vi "disdrometer_distrubitons.vi"(10 "Spectrum Vector":dbl[](array[numeric])=[1.0, 2.0, 3.0, 4.0, 5.0, 6.0, 7.0, 8.0, 9.0, 10.0, 11.0, 12.0]) -> (0 "Velocity Distribution":dbl[](array[numeric]), 1 "Diameter Distribution":dbl[](array[numeric]), 2 "Distribution Matrix":dbl[][](array[numeric]))   [LabVIEW 2018]
doc: "Separates disdrometer spectrum data into a diameter distribution array and a speed distribution array."
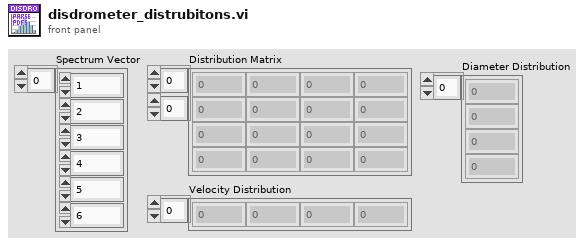
[diagram p1: front panel]
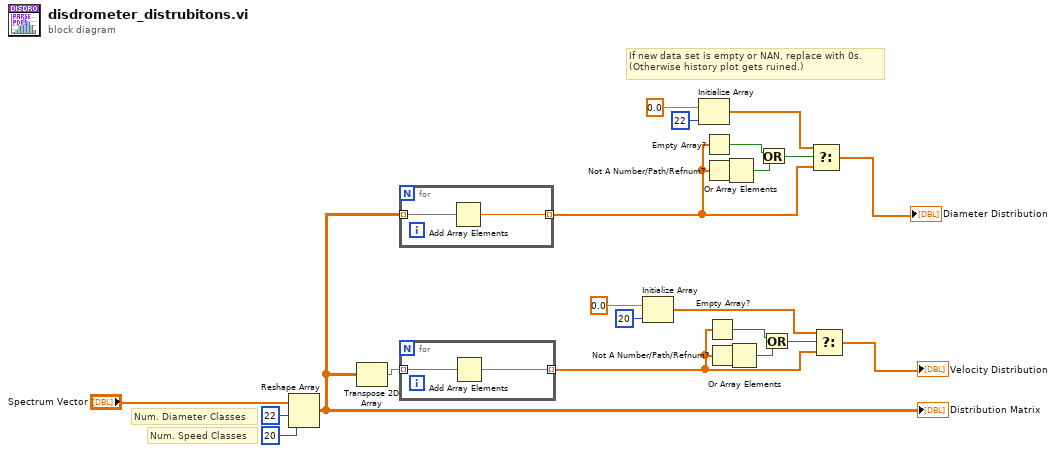
[diagram p0: block diagram]
diagram:
  # "If new data set is empty or NAN, replace with 0s.\n(Otherwise history plot gets ruined.)"
  # "Num. Speed Classes"
  # "Num. Diameter Classes"
  n1 = Reshape Array("Spectrum Vector", 22 ("dimension size"), 20 ("dimension size")) -> (w19:dbl[][])
  "Distribution Matrix" <- w19
  n2 = Transpose 2D Array(2D array=w19) -> (transposed array=w21:dbl[][])
  n3 = for {
    tunnel: w19 -> [w25] mode=indexing
    tunnel: [w24] -> w9 mode=indexing
    n4 = Add Array Elements(numeric array=w25) -> (sum=w24:dbl)
  }
  n5 = for {
    tunnel: w21 -> [w27] mode=indexing
    tunnel: [w26] -> w3 mode=indexing
    n6 = Add Array Elements(numeric array=w27) -> (sum=w26:dbl)
  }
  n7 = Initialize Array(0.0, 20 ("dimension size")) -> (w1:dbl[])
  n8 = Initialize Array(0.0, 22 ("dimension size")) -> (w12:dbl[])
  n9 = Empty Array?(array=w9) -> (empty?=w14:bool)
  n10 = Not A Number/Path/Refnum?(number/path/refnum=w9) -> (NaN/Path/Refnum?=w13:bool[])
  n11 = Empty Array?(array=w3) -> (empty?=w4:bool)
  n12 = Not A Number/Path/Refnum?(number/path/refnum=w3) -> (NaN/Path/Refnum?=w5:bool[])
  n13 = Or Array Elements(Boolean array=w13) -> (logical OR=w10:bool)
  n14 = Or Array Elements(Boolean array=w5) -> (logical OR=w7:bool)
  n15 = Or(x=w14, y=w10) -> (x .or. y?=w11:bool)
  n16 = Or(x=w4, y=w7) -> (x .or. y?=w6:bool)
  n17 = Select(t=w12, s=w11, f=w9) -> (s? t:f=→"Diameter Distribution":dbl[])
  n18 = Select(t=w1, s=w6, f=w3) -> (s? t:f=→"Velocity Distribution":dbl[])
